vi "select threat level.vi"(11 "input cluster":T1) -> (1 "Red":bool, 2 "Orange":bool, 3 "Yellow":bool)   [LabVIEW 2011]
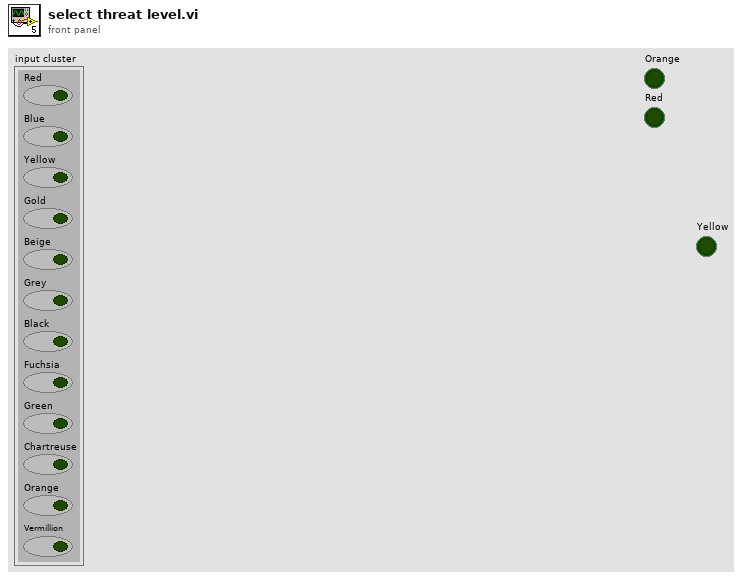
[diagram p1: front panel]
types:
  T1 = cluster{"Red":bool, "Blue":bool, "Yellow":bool, "Gold":bool, "Beige":bool, "Grey":bool, "Black":bool, "Fuchsia":bool, "Green":bool, "Chartreuse":bool, "Orange":bool, "Vermillion":bool}
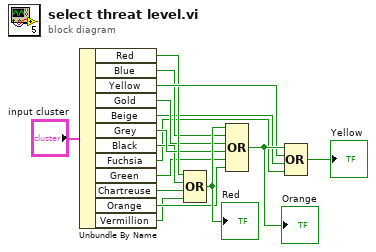
[diagram p0: block diagram]
diagram:
  n1 = Unbundle By Name("input cluster") -> ("Red"=w11:bool, "Blue"=w10:bool, "Yellow"=w12:bool, "Gold"=w9:bool, "Beige"=w8:bool, "Grey"=w7:bool, "Black"=w6:bool, "Fuchsia"=w5:bool, "Green"=w4:bool, "Chartreuse"=w3:bool, "Orange"=w2:bool, "Vermillion"=w1:bool)
  n2 = Compound Arithmetic op=OR(w11, w6, w3, w1) -> (w14:bool)
  "Red" <- w14
  n3 = Compound Arithmetic op=OR(w14, w10, w9, w7, w4, w2) -> (w13:bool)
  "Orange" <- w13
  n4 = Compound Arithmetic op=OR(w13, w12, w8, w5) -> (→"Yellow":bool)
